vi "example_02_multiple_plot.vi"() -> ()   [LabVIEW 2015, in "lv-graph-global.lvlib"]
uses:
  lv-graph-global.lvlib
  _controls/store_method.ctl
  _controls/configuration.ctl
  advanced/write-point.vi
  advanced/read-data.vi
  <userlib>/antonio-alexander/lv-graph/public/advanced/build_graph-multiple_axis.vi
  <userlib>/antonio-alexander/lv-graph/lv-graph.lvlib
panel:
  in  "store_method":T1=enum."grow"
  in  "number_of_rows":i32=1000
  in  "data_rate_ms_plot_2":u32=10
  in  "clear":bool
  out "multiple_x_axis":T2(graph)
  in  "data_rate_ms_plot_1":u32=20
  in  "refresh_rate_ms":u32=250
  in  "stop":bool
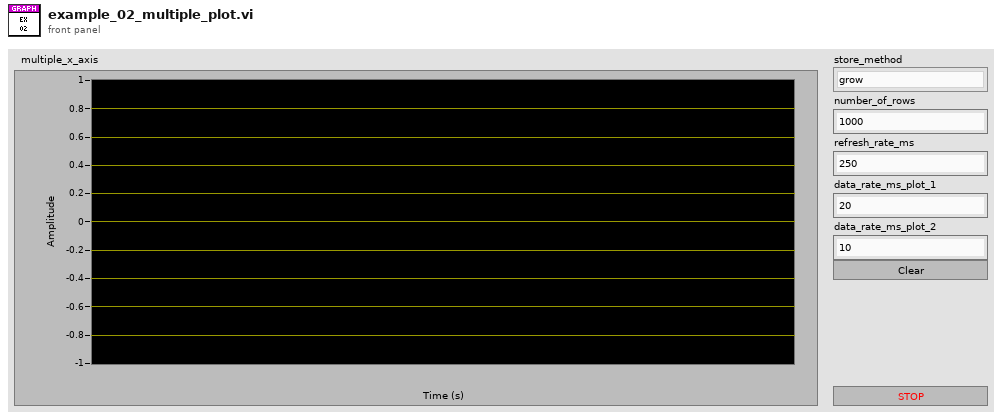
[diagram p1: front panel]
types:
  T1 = typedef "lv-graph-global.lvlib/store_method.ctl" = enum16{"<store_method>", "fixed", "grow"}
  T2 = cluster{"Time [] out":dbl[], "Data[][] out":dbl[]}[]
  T3 = enum8{"Enabled", "Disabled", "Disabled and Grayed Out"}
  T4 = typedef "lv-graph-global.lvlib/configuration.ctl" = cluster{"store_method":T1, "rows":i32, "columns":i32}
  T5 = cluster{"x_scale_maximum":dbl, "x_scale_minimum":dbl, "y_scale_maximum":dbl, "y_scale_minimum":dbl}
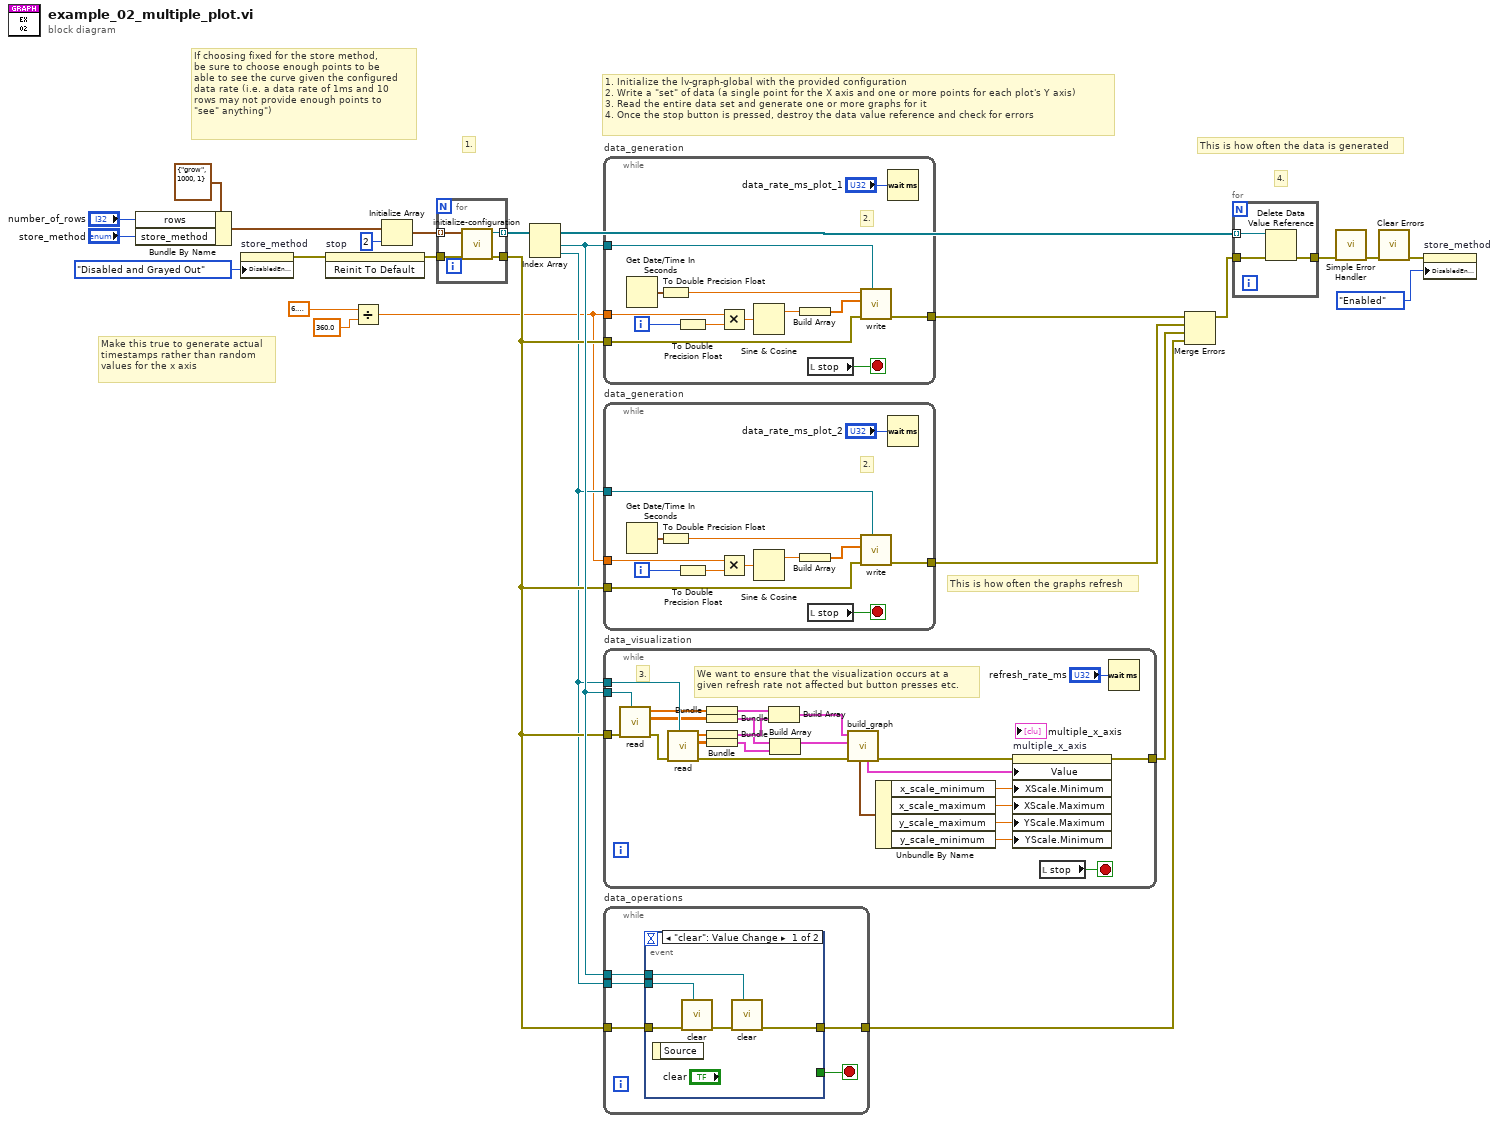
[diagram p0: block diagram]
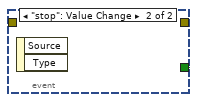
[diagram p2: hidden frame]
diagram:
  # "4."
  # "1."
  # "Make this true to generate actual\ntimestamps rather than random \nvalues for the x axis"
  # "This is how often the data is generated"
  # "This is how often the graphs refresh"
  # "If choosing fixed for the store method,\nbe sure to choose enough points to be\nable to see the curve given the configured\ndata rate (i.e. a data rate of 1ms and 10\nrows may not provide enough points to\n\"see\" anything\")"
  # "1. Initialize the lv-graph-global with the provided configuration\n2. Write a \"set\" of data (a single point for the X axis and one or more points for each plot's Y axis)\n3. Read the entire data set and generate one or more graphs for it\n4. Once the stop button is pressed, destroy the data value reference and check for errors"
  n1 = Bundle By Name(cluster=T4 {"store_method"=enum."grow", "rows"=1000, "columns"=1} ("configuration"), "rows"="number_of_rows", "store_method"="store_method") -> (w9:T4)
  n2 = property on="store_method" class="Enum (strict)"("DisabledEnum"=T3."Disabled and Grayed Out" ("Disabled")) -> (error out=w2:errorcluster)  [unwired: 2 in, 1 out]
  n3 = invoke on="stop" class="Bool (strict)" method="Reinit To Default"(error in=w2) -> (error out=w20:errorcluster)  [unwired: 2 in, 2 out]
  n4 = Divide(x=6.283185307179586, y=360.0) -> (x/y=w6:dbl)
  n5 = Initialize Array(w9, 2 ("dimension size")) -> (w12:T4[])
  n6 = for {
    tunnel: w12 -> [w29] mode=indexing
    tunnel: [w26] -> w16 mode=indexing
    tunnel: w20 -> [w28]
    tunnel: [w27] -> w14
    n7 = call "initialize-configuration.vi"("error in (no error)"=w28, "configuration"=w29) -> ("error out"=w27:errorcluster, "dvr"=w26:refnum<data-value>)  [unwired: 8 in]
  }
  n8 = Index Array(array=w16) -> (element #1=w17:refnum<data-value>, element #2=w13:refnum<data-value>)  [unwired: 2 in]
  n9 = while "data_generation" {
    tunnel: w14 -> [w34]
    tunnel: [w33] -> w25
    tunnel: w17 -> [w31]
    tunnel: w6 -> [w30]
    i -> [w40]
    stop <- w41 stop-if-true
    # "2."
    n10 = Get Date/Time In Seconds() -> (seconds since 1Jan1904=w42:timestamp)
    n11 = To Double Precision Float(number=w42) -> (double precision float=w38:dbl)
    n12 = To Double Precision Float(number=w40) -> (double precision float=w37:dbl)
    n13 = Multiply(x=w30, y=w37) -> (x*y=w36:dbl)
    n14 = Sine & Cosine(0:w36) -> (1:w35:dbl)  [unwired: 1 out]
    n15 = Build Array(w35) -> (w32:dbl[])
    n16 = local read "stop"() -> (w41:bool)
    n17 = call-poly "write.vi"("dvr"=w31, "error in (no error)"=w34, "y_axis"=w32, "x_axis"=w38) -> ("error out"=w33:errorcluster)  [unwired: 6 in, 1 out]
    n18 = Wait (ms)(milliseconds to wait="data_rate_ms_plot_1") -> ()  [unwired: 1 out]
  }
  n19 = while "data_generation" {
    tunnel: w14 -> [w48]
    tunnel: [w47] -> w15
    tunnel: w13 -> [w45]
    tunnel: w6 -> [w44]
    i -> [w53]
    stop <- w54 stop-if-true
    # "2."
    n20 = Get Date/Time In Seconds() -> (seconds since 1Jan1904=w55:timestamp)
    n21 = To Double Precision Float(number=w55) -> (double precision float=w51:dbl)
    n22 = To Double Precision Float(number=w53) -> (double precision float=w50:dbl)
    n23 = Multiply(x=w44, y=w50) -> (x*y=w49:dbl)
    n24 = Sine & Cosine(0:w49) -> (1:w43:dbl)  [unwired: 1 out]
    n25 = Build Array(w43) -> (w46:dbl[])
    n26 = local read "stop"() -> (w54:bool)
    n27 = call-poly "write.vi"("dvr"=w45, "error in (no error)"=w48, "y_axis"=w46, "x_axis"=w51) -> ("error out"=w47:errorcluster)  [unwired: 6 in, 1 out]
    n28 = Wait (ms)(milliseconds to wait="data_rate_ms_plot_2") -> ()  [unwired: 1 out]
  }
  n29 = while "data_visualization" {
    tunnel: w14 -> [w78]
    tunnel: w17 -> [w70]
    tunnel: [w68] -> w18
    tunnel: w13 -> [w67]
    stop <- w69 stop-if-true
    # "We want to ensure that the visualization occurs at a\ngiven refresh rate not affected but button presses etc."
    # "3."
    n30 = call-poly "read.vi"("dvr"=w70, "error in (no error)"=w78) -> ("error out"=w80:errorcluster, "y_axis"=w65:dbl[][], "x_axis"=w66:dbl[])  [unwired: 6 in, 1 out]
    n31 = call-poly "read.vi"("dvr"=w67, "error in (no error)"=w80) -> ("error out"=w56:errorcluster, "y_axis"=w63:dbl[][], "x_axis"=w64:dbl[])  [unwired: 6 in, 1 out]
    n32 = Bundle("x_axis"=w66) -> (w62:cluster{"x_axis":dbl[]})  [unwired: 1 in]
    n33 = Bundle("y_axis"=w65) -> (w59:cluster{"y_axis":dbl[][]})  [unwired: 1 in]
    n34 = Bundle("x_axis"=w64) -> (w61:cluster{"x_axis":dbl[]})  [unwired: 1 in]
    n35 = Bundle("y_axis"=w63) -> (w60:cluster{"y_axis":dbl[][]})  [unwired: 1 in]
    n36 = Build Array(w62, w61) -> (w58:cluster{"x_axis":dbl[]}[])
    n37 = Build Array(w59, w60) -> (w57:cluster{"y_axis":dbl[][]}[])
    n38 = call-poly <userlib>:"build_graph.vi"("error in (no error)"=w56, "y_axis"=w57, "x_axis"=w58) -> ("error out"=w73:errorcluster, "graph_data"=w71:cluster{dbl[], dbl[]}[], "scale_range"=w72:T5)  [unwired: 6 in]
    n39 = Unbundle By Name(w72) -> ("x_scale_minimum"=w75:dbl, "x_scale_maximum"=w74:dbl, "y_scale_maximum"=w76:dbl, "y_scale_minimum"=w77:dbl)
    n40 = property on="multiple_x_axis" class="XYGraph (strict)"(error in=w73, "Value"=w71, "XScale.Minimum"=w75, "XScale.Maximum"=w74, "YScale.Maximum"=w76, "YScale.Minimum"=w77) -> (error out=w68:errorcluster)  [unwired: 1 in, 1 out]
    n41 = local read "stop"() -> (w69:bool)
    n42 = Wait (ms)(milliseconds to wait="refresh_rate_ms") -> ()  [unwired: 1 out]
  }
  n43 = while "data_operations" {
    tunnel: w14 -> [w85]
    tunnel: w17 -> [w84]
    tunnel: [w82] -> w19
    tunnel: w13 -> [w81]
    stop <- w83 stop-if-true
    n44 = event shown="[0] \"clear\": Value Change" {
      selector: _ -> [_ _]
      dyn-events: _ -> [_ _]
      timeout: _ -> [_ _]
      tunnel: w85 -> [w90 _]
      tunnel: w84 -> [w87 _]
      tunnel: [_ TRUE] -> w83
      tunnel: [w88 _] -> w82
      tunnel: w81 -> [w86 _]
      event "clear": Value Change {
        n45 = event-data() -> ()  [unwired: 1 in, 1 out]
        n46 = call "clear.vi"("dvr"=w86, "error in (no error)"=w90) -> ("error out"=w89:errorcluster)  [unwired: 9 in]
        n47 = call "clear.vi"("dvr"=w87, "error in (no error)"=w89) -> ("error out"=w88:errorcluster)  [unwired: 9 in]
      }
      event "stop": Value Change {
        n48 = event-data() -> ()  [unwired: 1 in, 2 out]
      }
    }
  }
  n49 = Merge Errors(w25, w15, w18, w19) -> (w24:errorcluster)
  n50 = for {
    tunnel: w16 -> [w92] mode=indexing
    tunnel: w24 -> [w94]
    tunnel: [w93] -> w21
    n51 = Delete Data Value Reference(data value reference=w92, error in=w94) -> (error out=w93:errorcluster)  [unwired: 1 out]
  }
  n52 = call <vilib>:"Simple Error Handler.vi"("error in (no error)"=w21) -> ("error out"=w5:errorcluster)  [unwired: 4 in, 4 out]
  n53 = call <vilib>:"Clear Errors.vi"("error in (no error)"=w5) -> ("error out"=w4:errorcluster)  [unwired: 5 in, 1 out]
  n54 = property on="store_method" class="Enum (strict)"(error in=w4, "DisabledEnum"=T3."Enabled" ("Disabled")) -> ()  [unwired: 1 in, 2 out]
